vi "Lesson_2.vi"() -> ()   [LabVIEW 2019]
uses:
  SignalTypeEnum.ctl
  StatesEnum.ctl
panel:
  in  "frequency (1)":dbl=1.0 format="%0.2f"
  in  "amplitude (1)":dbl=1.0 format="%0.2f"
  in  "signal type":T1
  in  "Stop Button":bool
  out "Waveform Chart":dbl(graph)=-0.8479582352014673
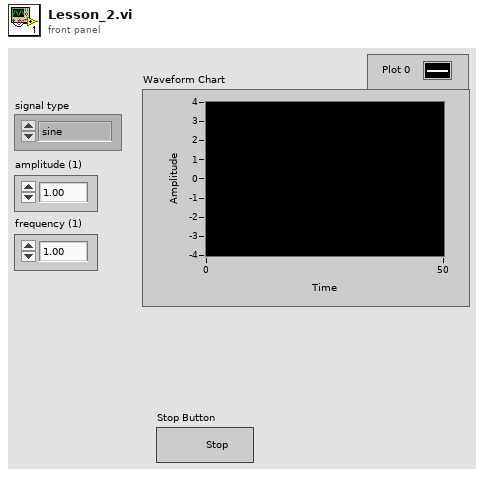
[diagram p1: front panel]
types:
  T1 = typedef "SignalTypeEnum.ctl" = enum16{"sine", "cosine", "triangle", "square"}
  T2 = typedef "StatesEnum.ctl" = enum16{"Clear Chart", "Acquire Data", "Wait on User Input", "Exit"}
  T3 = cluster{"signal type":T1, "amplitude (1)":dbl, "frequency (1)":dbl}
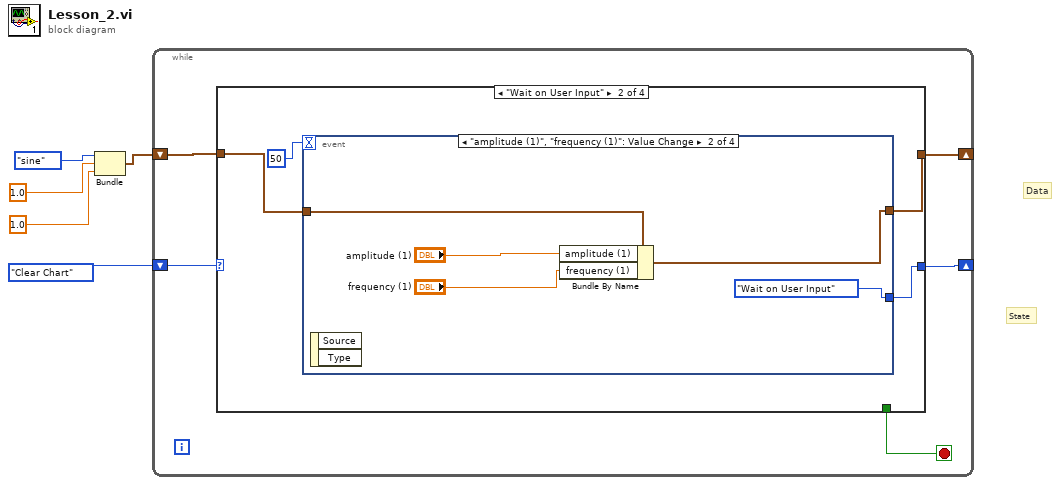
[diagram p0: block diagram]
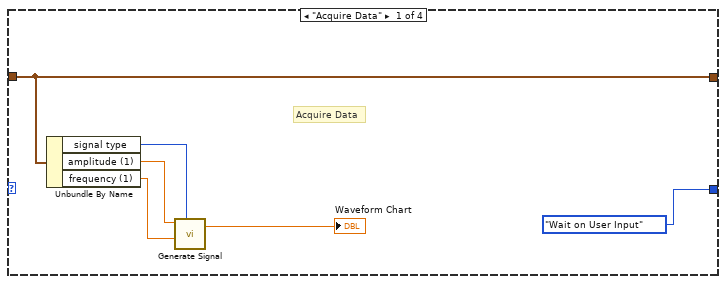
[diagram p2: hidden frame]
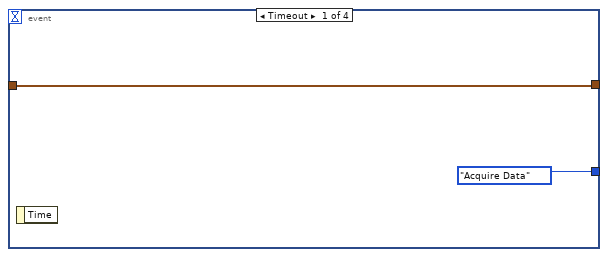
[diagram p3: hidden frame]
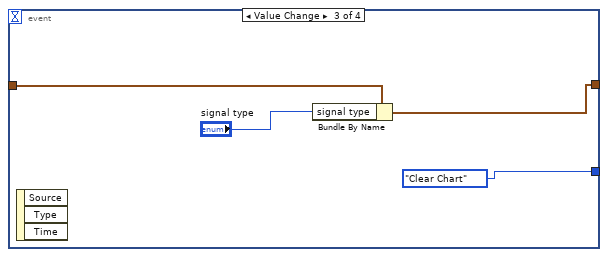
[diagram p4: hidden frame]
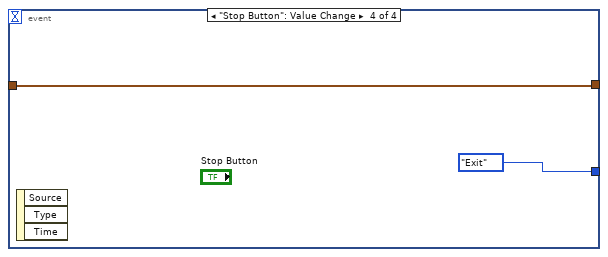
[diagram p5: hidden frame]
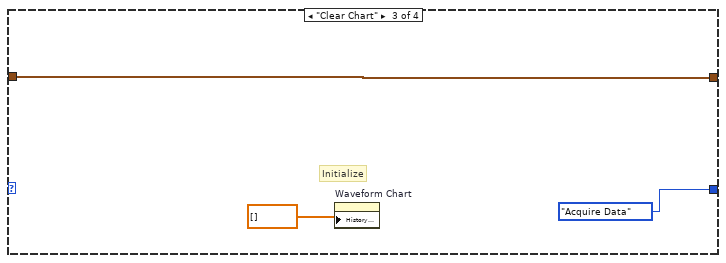
[diagram p6: hidden frame]
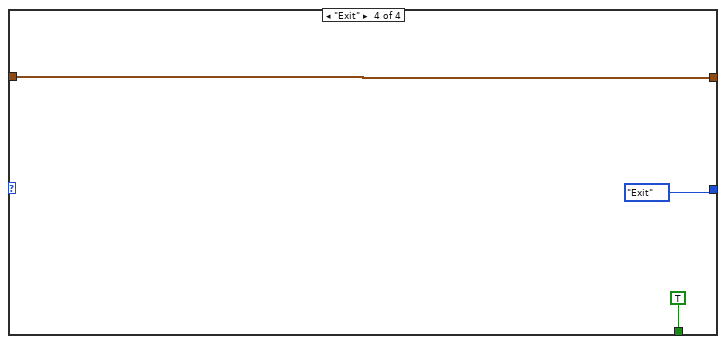
[diagram p7: hidden frame]
diagram:
  # "State"
  # "Data"
  n1 = Bundle("signal type"=SignalTypeEnum."sine", "amplitude (1)"=1.0, "frequency (1)"=1.0) -> (w2:T3)  [unwired: 1 in]
  n2 = while {
    shift-right: [w9] -> _
    shift-left: w2 -> [w8]
    shift-right: [w7] -> _
    shift-left: StatesEnum."Clear Chart" -> [w10]
    stop <- w6 stop-if-true
    n3 = case shown="\"Wait on User Input\"" w10 {
      tunnel: [w14 w18 w34 w39] -> w9
      tunnel: w8 -> [w14 w20 w34 w39]
      tunnel: [StatesEnum."Wait on User Input" w19 StatesEnum."Acquire Data" StatesEnum."Exit"] -> w7
      tunnel: [_ _ _ TRUE ("Stop Button")] -> w6
      frame "Acquire Data" {
        # "Acquire Data"
        n4 = Unbundle By Name(w14) -> ("signal type"=w13:T1, "amplitude (1)"=w12:dbl, "frequency (1)"=w11:dbl)
        n5 = call "Generate Signal.vi"("signal type"=w13, "frequency (1)"=w11, "amplitude (1)"=w12) -> ("wave form"=→"Waveform Chart":dbl)  [unwired: 7 in, 1 out]
      }
      frame "Wait on User Input" {
        n6 = event shown="[1] \"amplitude (1)\", \"frequency (1)\": Value Change" {
          selector: _ -> [_ _ _ _]
          dyn-events: _ -> [_ _ _ _]
          timeout: 50 -> [_ _ _ _]
          tunnel: w20 -> [w22 w26 w29 w32]
          tunnel: [StatesEnum."Acquire Data" StatesEnum."Wait on User Input" StatesEnum."Clear Chart" StatesEnum."Exit"] -> w19
          tunnel: [w22 w27 w28 w32] -> w18
          event Timeout {
            n7 = event-data() -> ()  [unwired: 1 in, 1 out]
          }
          event "amplitude (1)", "frequency (1)": Value Change {
            n8 = event-data() -> ()  [unwired: 1 in, 2 out]
            n9 = Bundle By Name(cluster=w26, "amplitude (1)"="amplitude (1)", "frequency (1)"="frequency (1)") -> (w27:T3)
          }
          event Value Change {
            n10 = event-data() -> ()  [unwired: 1 in, 3 out]
            n11 = Bundle By Name(cluster=w29, "signal type"="signal type") -> (w28:T3)
          }
          event "Stop Button": Value Change {
            n12 = event-data() -> ()  [unwired: 1 in, 3 out]
          }
        }
      }
      frame "Clear Chart" {
        # "Initialize"
        n13 = property on="Waveform Chart" class="WFChart (strict)"("History Data"=dbl[] []) -> ()  [unwired: 2 in, 2 out]
      }
      frame "Exit" {
      }
    }
  }
